vi "index to type.vi"(11 "I32":i32) -> (3 "type":T1)   [LabVIEW 2013, in "tag bus.lvlib" / "tag descriptor.lvclass"]
doc: "A helper function which converts between a standard indexing terminal (I32) and the type enum provided by the framework (U16)."
uses:
  tag descriptor.lvclass
  Data Type.ctl
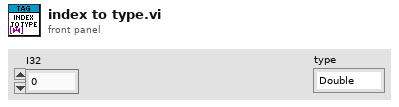
[diagram p1: front panel]
types:
  T1 = typedef "tag bus.lvlib/tag descriptor.lvclass/Data Type.ctl" = enum16{"Double", "Single", "I64", "I32", "I16", "I8", "U64", "U32", "U16", "U8", "Boolean", "String", "Array of Double", "Array of Single", "Array of I64", "Array of I32", "Array of I16", "Array of I8", "Array of U64", "Array of U32", "Array of U16", "Array of U8", "Array of Boolean", "Array of String"}
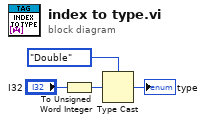
[diagram p0: block diagram]
diagram:
  n1 = To Unsigned Word Integer(number="I32") -> (unsigned 16bit integer=w4:u16)
  n2 = Type Cast(type=Data_Type."Double" ("Data Type"), x=w4) -> (*(type *) &x=→"type":T1)
